vi "CloseApp.vi"(8 "error in (no error)":errorcluster, 11 "Application Data":T1) -> (0 "error out":errorcluster)   [LabVIEW 2019]
uses:
  Typedefs/#cluster_ApplicationData.ctl
  <vilib>/ActorFramework/Message Enqueuer/Message Enqueuer.lvclass
  Typedefs/Acquisition Thread/#cluster_AcqQueueData.ctl
  Typedefs/Acquisition Thread/#enum_AcquisitionTask.ctl
  Typedefs/Saving Thread/#cluster_SavingQueueData.ctl
  Typedefs/Saving Thread/#enum_SavingTask.ctl
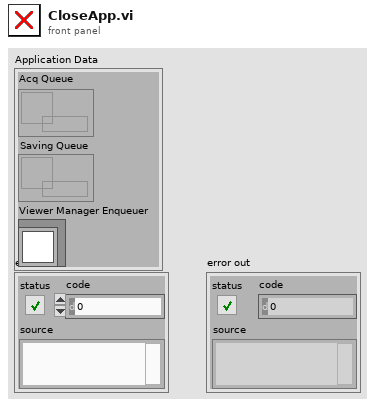
[diagram p1: front panel]
types:
  T1 = typedef "#cluster_ApplicationData.ctl" = cluster{"Acq Queue":refnum<queue>, "Saving Queue":refnum<queue>, "Viewer Manager Enqueuer":refnum<class "Message Enqueuer.lvclass">}
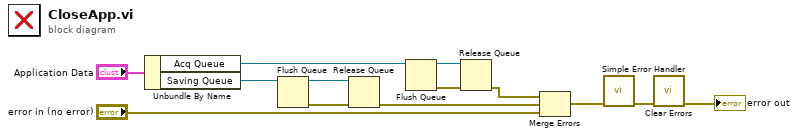
[diagram p0: block diagram]
diagram:
  n1 = Unbundle By Name("Application Data") -> ("Acq Queue"=w2:refnum<queue>, "Saving Queue"=w6:refnum<queue>)
  n2 = Flush Queue(queue=w6) -> (queue out=w5:refnum<queue>, error out=w4:errorcluster)  [unwired: 1 in, 1 out]
  n3 = Release Queue(queue=w5, error in (no error)=w4) -> (error out=w11:errorcluster)  [unwired: 1 in, 2 out]
  n4 = Flush Queue(queue=w2) -> (queue out=w1:refnum<queue>, error out=w3:errorcluster)  [unwired: 1 in, 1 out]
  n5 = Release Queue(queue=w1, error in (no error)=w3) -> (error out=w12:errorcluster)  [unwired: 1 in, 2 out]
  n6 = Merge Errors(w12, w11, "error in (no error)") -> (w9:errorcluster)
  n7 = call <vilib>:"Simple Error Handler.vi"("error in (no error)"=w9) -> ("error out"=w8:errorcluster)  [unwired: 4 in, 4 out]
  n8 = call <vilib>:"Clear Errors.vi"("error in (no error)"=w8) -> ("error out"=→"error out":errorcluster)  [unwired: 5 in, 1 out]
